vi "Autonomous Independent.vi"() -> ()   [LabVIEW 2015]
doc: "This VI is called when autonomous begins, and will automatically be terminated when autonomous ends. You can carry out timed or sensor driven robot movement independently without needing to return to the caller."
uses:
  <vilib>/Rock Robotics/WPI/CAN/TalonSRX/WPI_CANTalonSRX_BrakeOverride.ctl
  <vilib>/Rock Robotics/WPI/Utilities/WPI_GetSetVariantRefNum.vi
  <vilib>/Rock Robotics/Network Tables/NT Read String.vi
  <vilib>/Rock Robotics/Network Tables/NT Write Numeric Array.vi
  <vilib>/Rock Robotics/Network Tables/NT Write Number.vi
  <vilib>/addons/control/pid/pid.llb/PID (DBL).vi
  Robot Global Data.vi
  <vilib>/Rock Robotics/Network Tables/NT Read Number.vi
  <vilib>/addons/control/pid/NI_PID_pid.lvlib
  navX Library v2/navX Library v2.lvlib
panel:
  out "Shooter Output":dbl(graph)
  in  "Shoot Gains":T1={"proportional gain (Kc)"=1.0, "integral time (Ti, min)"=0.01, "derivative time (Td, min)"=0.0} {"derivative time (Td, min)" format="%.3f"; "integral time (Ti, min)" format="%.3f"; "proportional gain (Kc)" format="%.3f"}
  out "RPM":dbl(graph)
  in  "RPM 2":dbl
  in  "RPM":dbl
  in  "Aiming Gains":T1={"proportional gain (Kc)"=1.0, "integral time (Ti, min)"=0.01, "derivative time (Td, min)"=0.0} {"derivative time (Td, min)" format="%.3f"; "integral time (Ti, min)" format="%.3f"; "proportional gain (Kc)" format="%.3f"}
  out "Yaw":dbl(graph)
  in  "Target Angle":dbl=30.0
  out "E1 Rate":dbl
  out "E2 Rate":dbl
  out "Yaw Display":dbl
  in  "Single Turn Gains":T1={"proportional gain (Kc)"=0.12, "integral time (Ti, min)"=0.0, "derivative time (Td, min)"=0.0} {"derivative time (Td, min)" format="%.3f"; "integral time (Ti, min)" format="%.3f"; "proportional gain (Kc)" format="%.3f"}
  in  "Yaw":T1={"proportional gain (Kc)"=0.2, "integral time (Ti, min)"=0.0, "derivative time (Td, min)"=0.0} {"derivative time (Td, min)" format="%.3f"; "integral time (Ti, min)" format="%.3f"; "proportional gain (Kc)" format="%.3f"}
  out "Right Motor Speed":dbl(graph)
  out "Left Motor Speed":dbl(graph)
  out "Right Motor":dbl(graph)
  out "Left Motor":dbl(graph)
  in  "Distance":dbl=120.0
  in  "Speed Gains":T1={"proportional gain (Kc)"=0.65, "integral time (Ti, min)"=0.001, "derivative time (Td, min)"=0.001} {"derivative time (Td, min)" format="%.3f"; "integral time (Ti, min)" format="%.3f"; "proportional gain (Kc)" format="%.3f"}
  out "E2 Dist":dbl
  out "E1 Dist":dbl
  # "Be sure to right-click and choose Data Operations>>Make Current Value default if you want to save the array values with the VI"
  # "Encoder Distance Traveled"
  # "Speed we are assigning the motors and Encoder Rate"
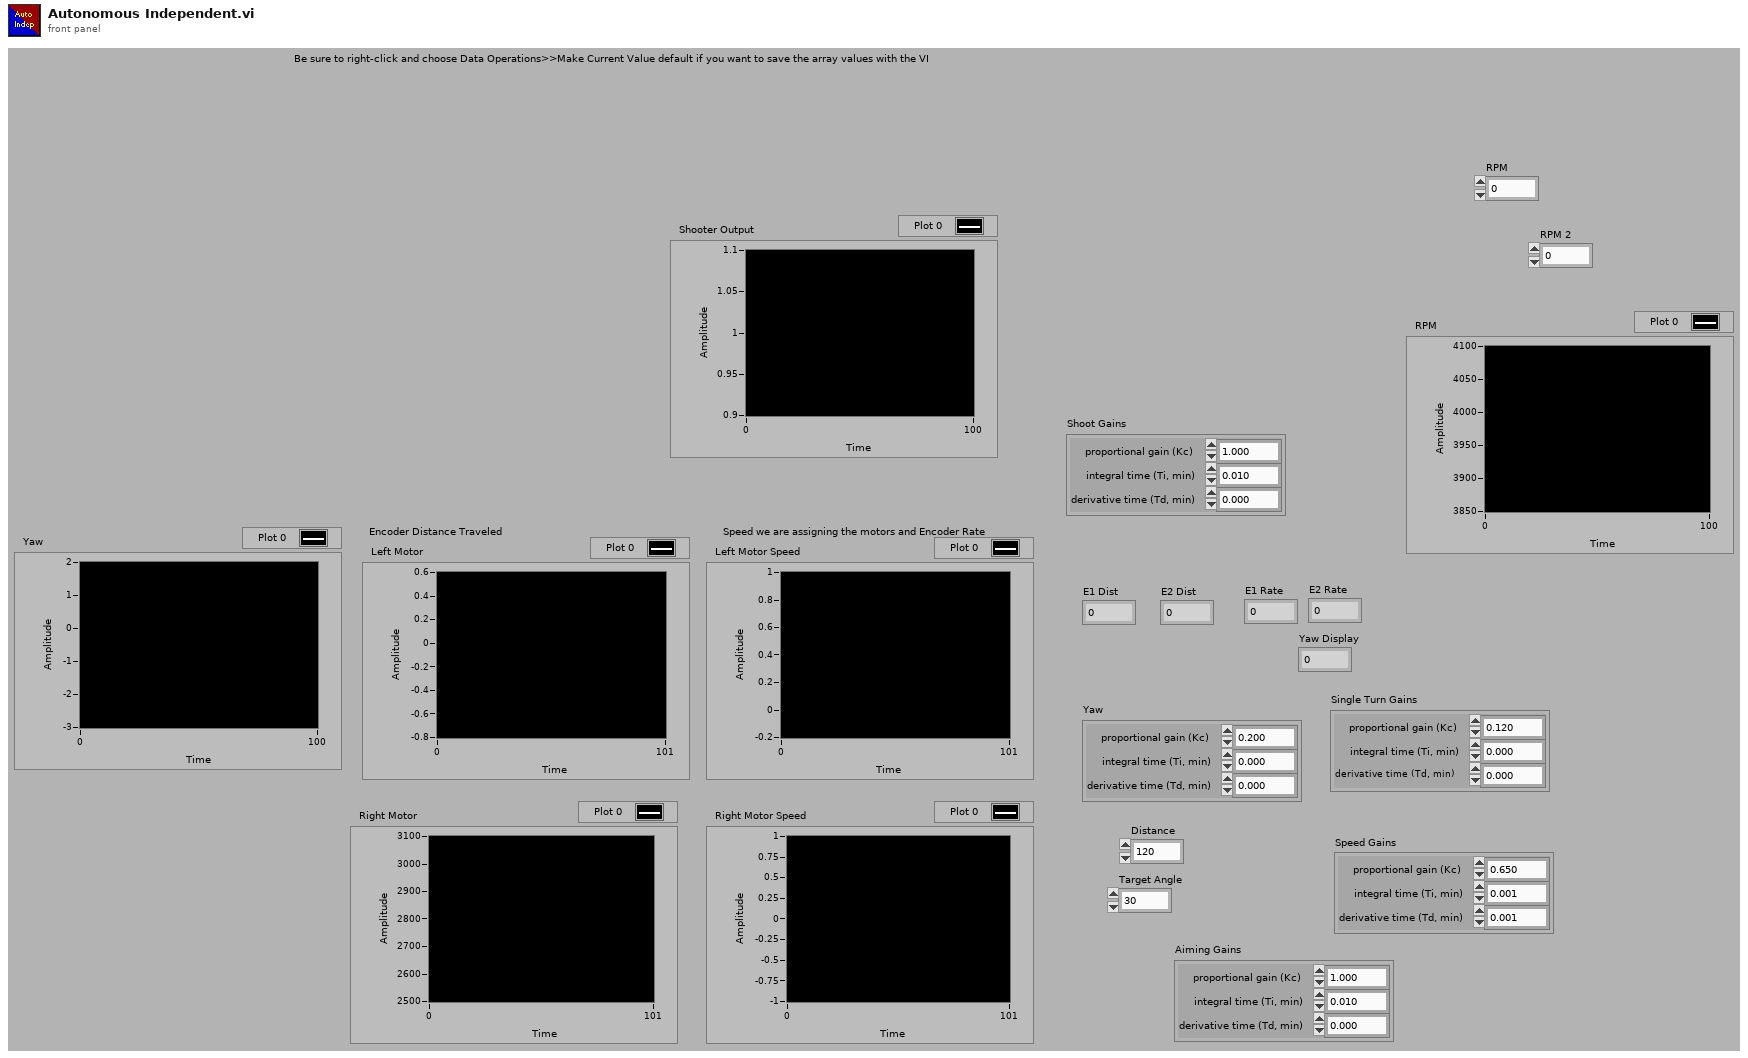
[diagram p1: front panel]
types:
  T1 = cluster{"proportional gain (Kc)":dbl, "integral time (Ti, min)":dbl, "derivative time (Td, min)":dbl}
  T2 = typedef "WPI_JoystickDevRef.ctl" = cluster{"Device":T3}
  T3 = typedef "WPI_JoystickDeviceEnum.ctl" = enum16{"USB 0", "USB 1", "USB 2", "USB 3", "USB 4", "USB 5"}
  T4 = typedef "WPI_CANTalonSRX_BrakeOverride.ctl" = enum8{"No Override", "Override to Coast", "Override to Brake"}
  T5 = typedef "navX Library v2.lvlib/Z900_navX_DeviceTypeDef.ctl" = cluster{"Interface":cluster{"Protocol":T6, "Update Rate (4Hz-60Hz)":u8, "navX Open TypeDef":variant}, "Notify Packet":refnum<notifier>, "Loop VI Refnum":refnum<vi>, "Ready to Close Occurrence Refnum":refnum<k4>}
  T6 = typedef "navX Library v2.lvlib/Z900_navX_ProtocolTypeDef.ctl" = enum16{"SERIAL", "I2C", "SPI"}
  T7 = typedef "WPI_EncoderDevRef.ctl" = cluster{"DevStatus":errorcluster, "EncoderIndex":T8, "CounterIndex":T9, "DistancePerCount":dbl, "Decoding Type":T10}
  T8 = typedef "FPGA_EncoderIdx.ctl" = enum8{"Enc 0", "Enc 1", "Enc 2", "Enc 3", "Enc 4", "Enc 5", "Enc 6", "Enc 7", "Invalid"}
  T9 = typedef "FPGA_CounterCtrSystemIndex.ctl" = enum8{"Ctr 0", "Ctr 1", "Ctr 2", "Ctr 3", "Ctr 4", "Ctr 5", "Ctr 6", "Ctr 7", "Invalid"}
  T10 = typedef "WPI_EncoderType.ctl" = enum16{"1x", "2x", "4x"}
  T11 = cluster{"Yaw":dbl, "Roll":dbl, "Pitch":dbl, "Heading":dbl, "Fused Heading":dbl}
  T12 = typedef "WPI_RobotDriveDevRef.ctl" = cluster{"DevStatus":errorcluster, "Motors[]":T13[], "Square Inputs":bool, "Max Output":dbl}
  T13 = typedef "WPI_MotorControlDeviceRef.ctl" = cluster{"DeviceStatus":errorcluster, "Type":T14, "PWM":cluster{"PWM Channel":T15, "DeadBand":T16}, "CAN":cluster{"Device Number":u8, "Control Mode":T17, "Semaphore":T18, "Max Vout":dbl, "TalonSRX Control Mode":T19}, "Invert":bool}
  T14 = typedef "WPI_MotorControlType.ctl" = enum16{"PWM", "CAN", "CANTalonSRX"}
  T15 = typedef "FPGA_DIOPWMChannel.ctl" = enum8{"PWM 0", "PWM 1", "PWM 2", "PWM 3", "PWM 4", "PWM 5", "PWM 6", "PWM 7", "PWM 8", "PWM 9", "PWM MXP 0", "PWM MXP 1", "PWM MXP 2", "PWM MXP 3", "PWM MXP 4", "PWM MXP 5", "PWM MXP 6", "PWM MXP 7", "PWM MXP 8", "PWM MXP 9", "Invalid"}
  T16 = typedef "WPI_PWMDeadband.ctl" = cluster{"Name":string, "maxPositivePwm":i32, "minPositivePwm":i32, "centerPwm":i32, "maxNegativePwm":i32, "minNegativePwm":i32, "angularRange":u16}
  T17 = typedef "WPI_CANJaguar_ControlMode.ctl" = enum8{"Percent VBus", "Current", "Speed", "Position", "Voltage"}
  T18 = typedef "Semaphore RefNum" = refnum<k1>
  T19 = typedef "WPI_CANTalonSRX_APIControlMode.ctl" = enum8{"Percent VBus", "Speed", "Position", "Slave", "Unchanged / Invalid", "Voltage Compensation", "Current", "Motion Profile"}
  T20 = typedef "WPI_CANTalonSRX_GlobalStatus.ctl" = cluster{"Applied Throttle":dbl, "Module Enabled":bool, "CAN Error":errorcluster, "Closed Loop Error":dbl, "Forward Limit Switch Closed":bool, "Reverse Limit Switch Closed":bool, "Sensor Position":dbl, "Sensor Velocity":dbl, "Current":dbl, "Sticky Fault - Over Temp":bool, "Sticky Fault - Under Voltage":bool, "Sticky Fault - Forward Limit":bool, "Sticky Fault - Reverse Limit":bool, "Sticky Fault - Forward Soft Limit":bool, "Sticky Fault - Reverse Soft Limit":bool, "Brake is Enabled":bool, "Encoder Position":dbl, "Encoder Velocity":dbl, "Encoder Index Count":dbl, "Encoder A Pin State":bool, "Encoder B Pin State":bool, "Encoder Index Pin State":bool, "Analog In":dbl, "Analog In Velocity":dbl, "Temperature (C)":dbl, "Battery Voltage":dbl, "Control 5 Is Supported":bool, "Current Profile Slot Select":dbl, "Pos Div 8":bool, "Vel Div 4":bool, "Pulse Width Position":i32, "Pulse Width Velocity":i32, "Pulse Width Rise To Rise (us)":i32, "Pulse Width Rise To Fall (us)":i32, "Mot Prof Active Is Under Run":bool, "Mot Prof Active Has Under Run":bool, "Mot Prof Active Is Last":bool, "Mot Prof Active Velocity Only":bool, "Mot Prof Active Is Valid":bool, "Mot Prof Buffer Is Full":bool, "Mot Prof Active Profile Slot Select":i32, "Mot Prof NextID":i32, "Mot Prof Count":i32, "Mot Prof Active Velocity":dbl, "Mot Prof Active Position":dbl, "Mot Prof Output Enable":i32}
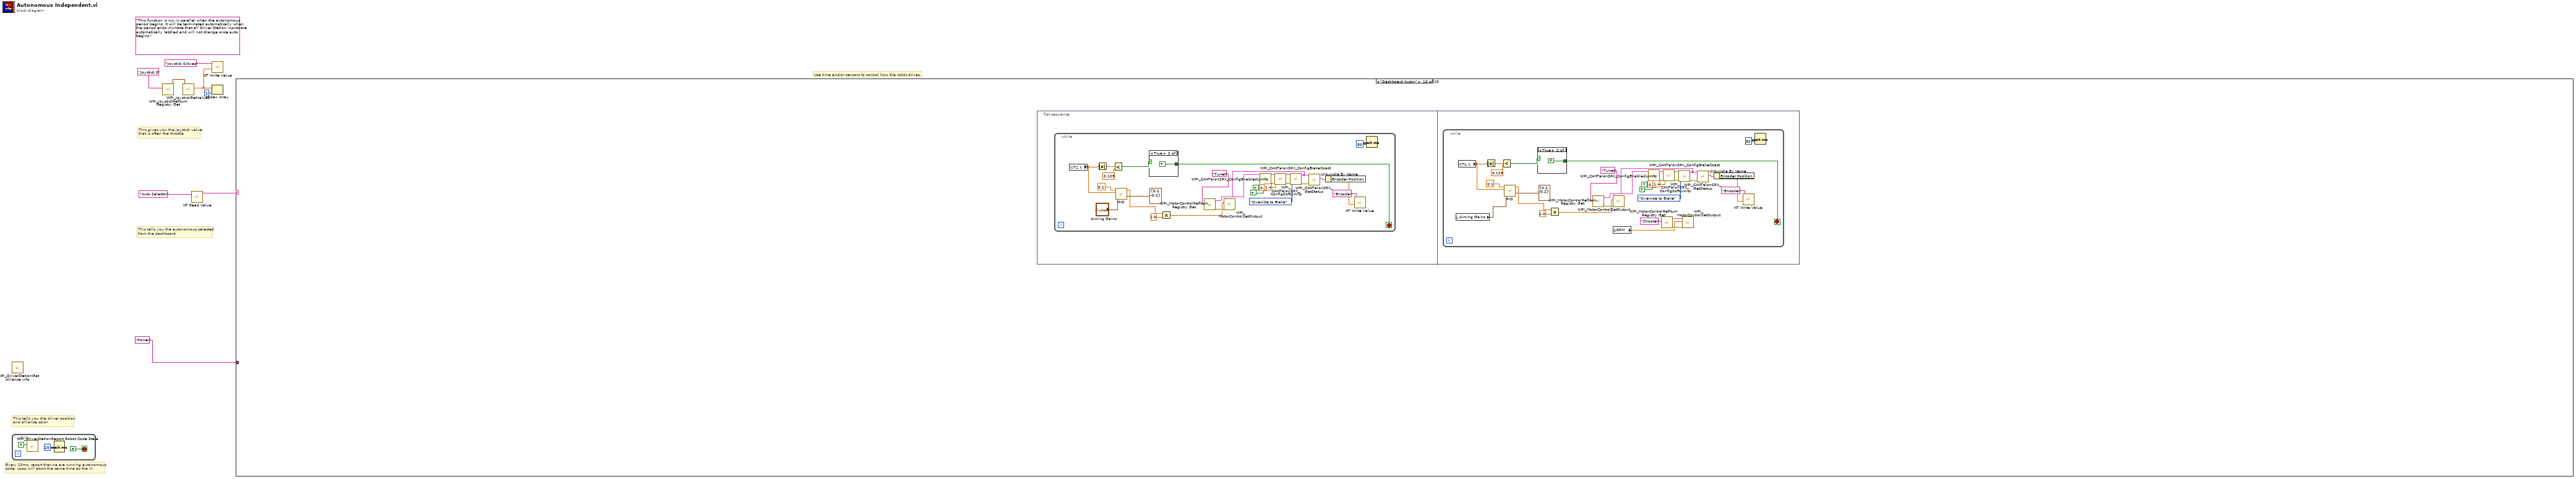
[diagram p0: block diagram]
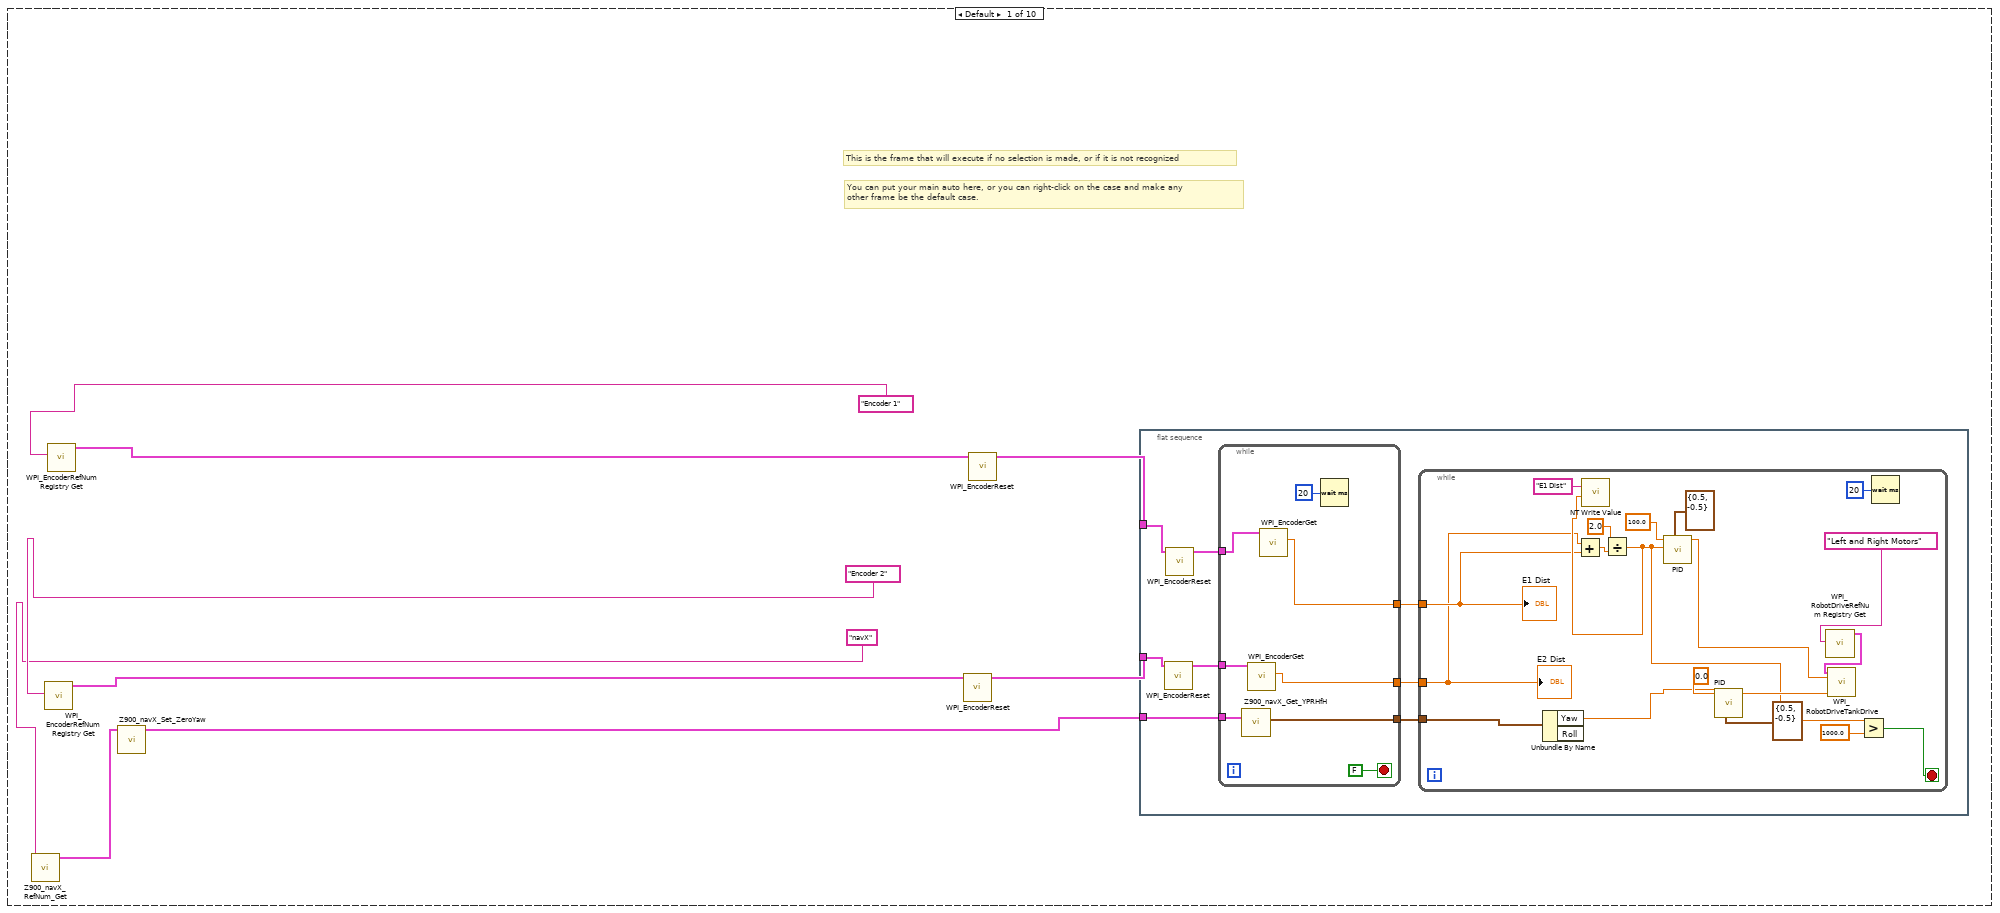
[diagram p2: hidden frame]
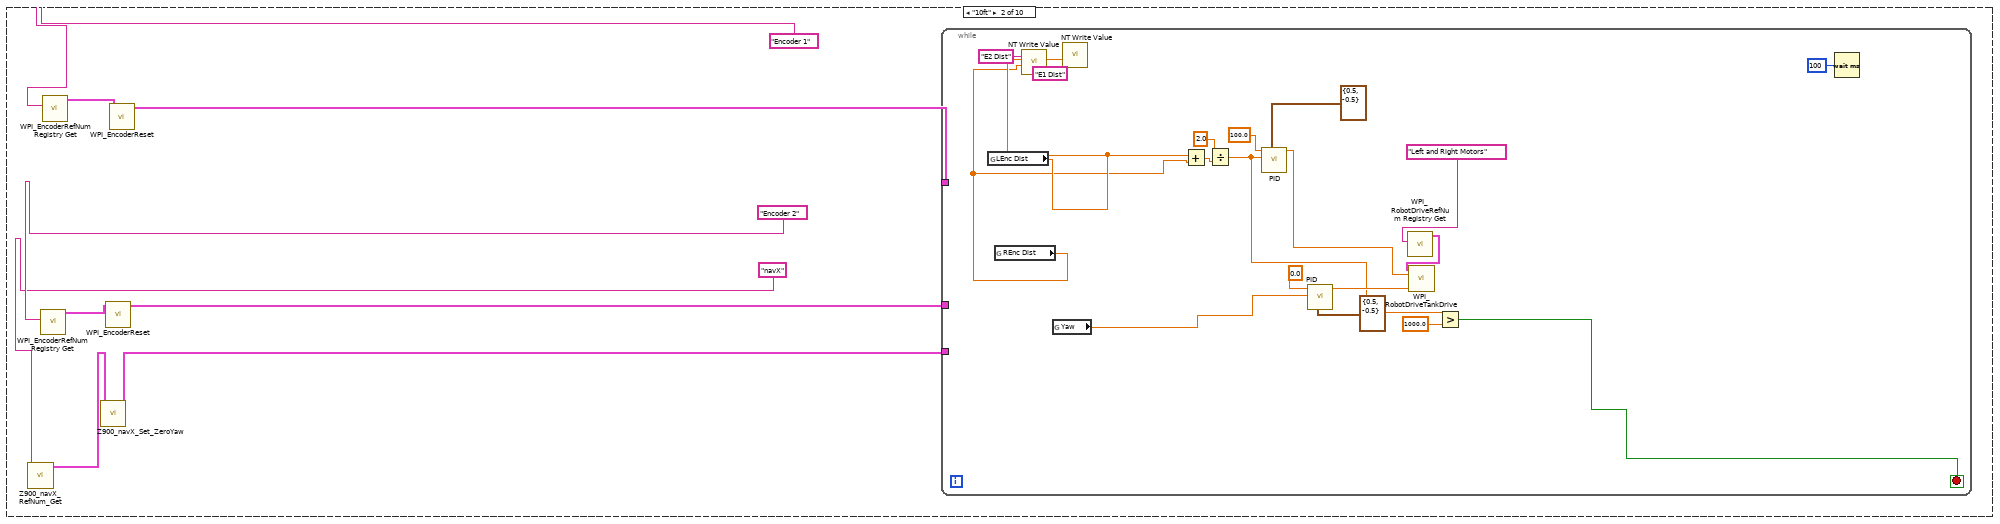
[diagram p3: hidden frame]
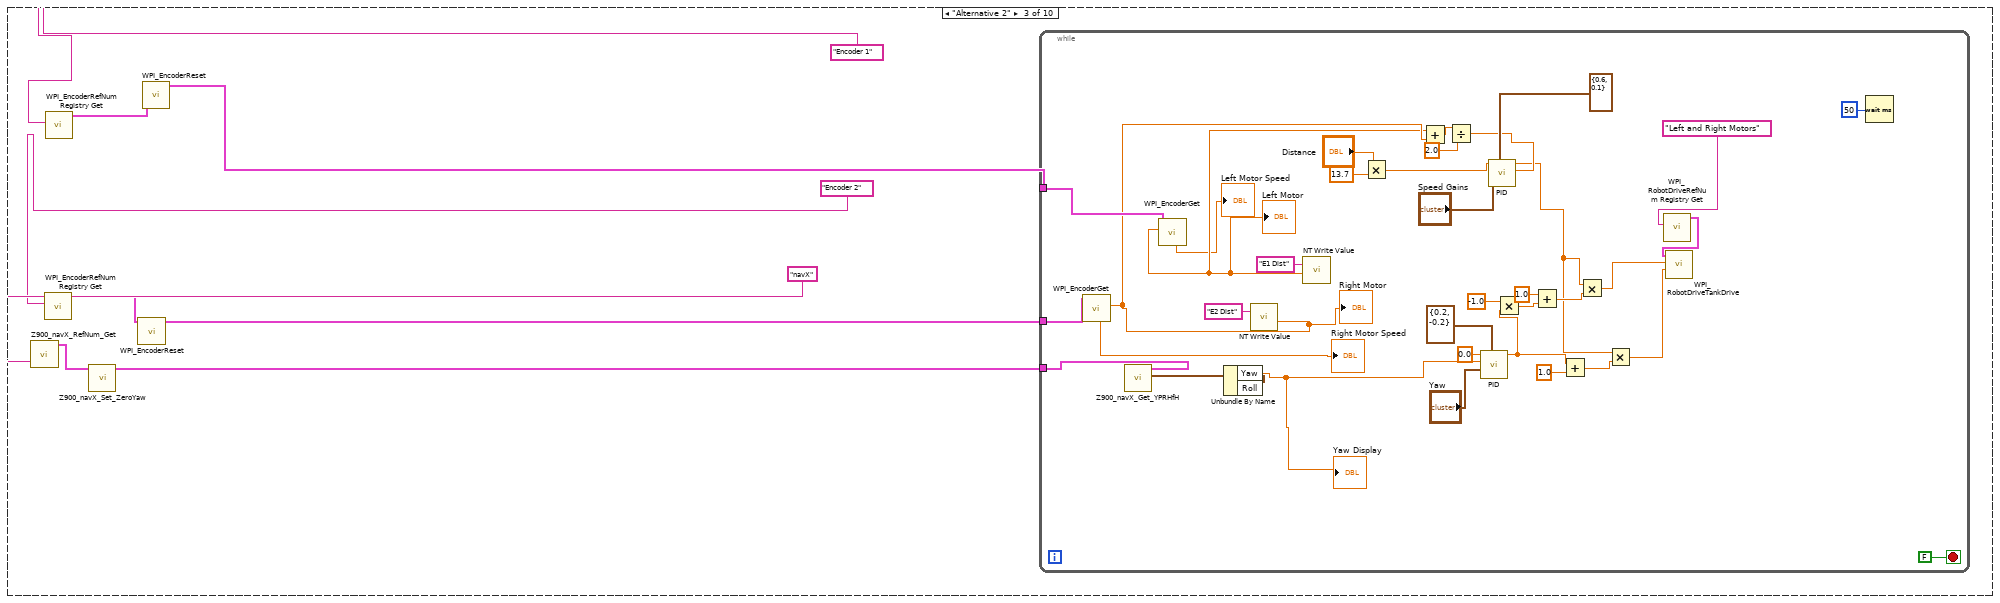
[diagram p4: hidden frame]
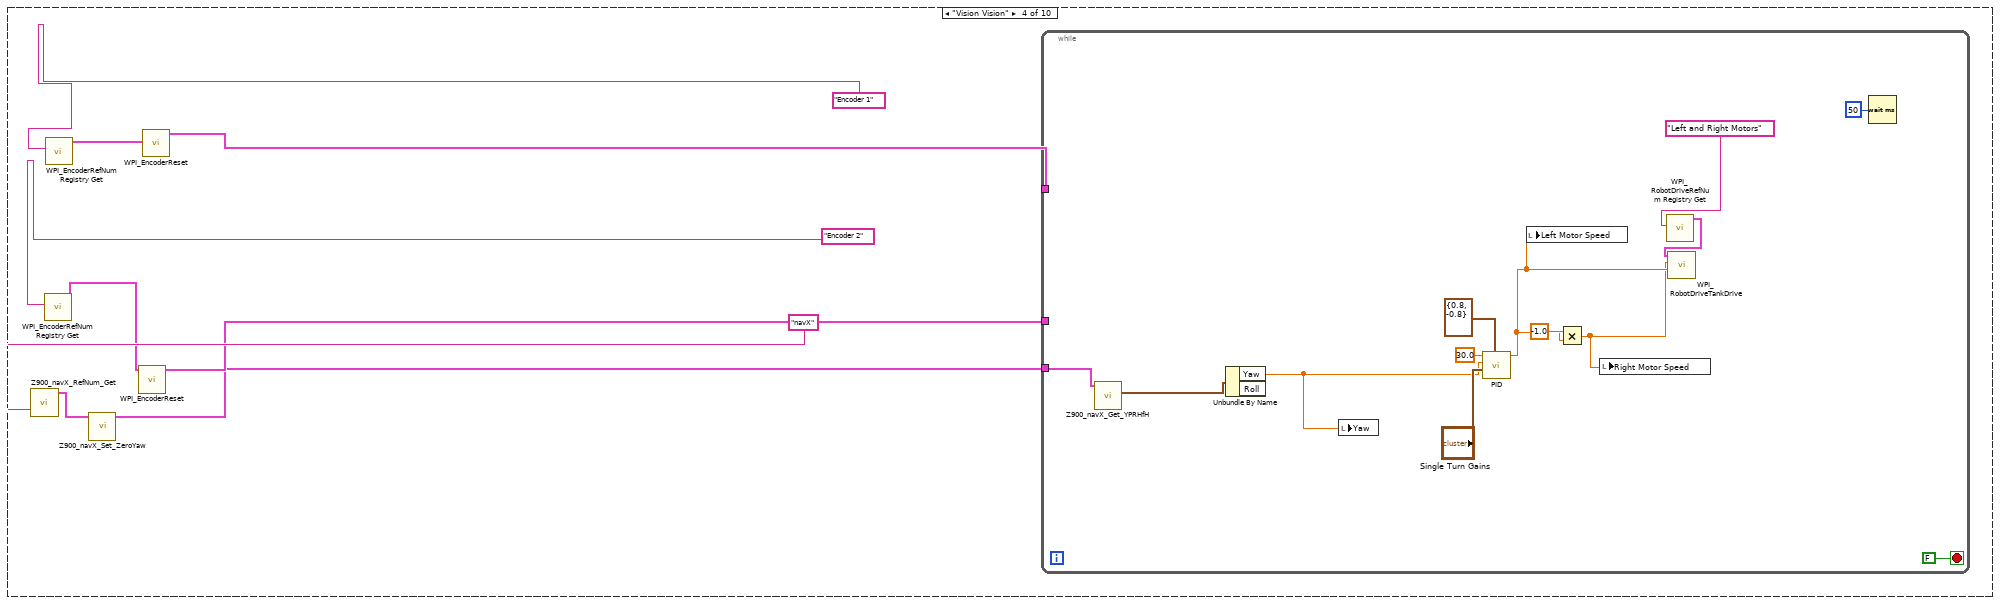
[diagram p5: hidden frame]
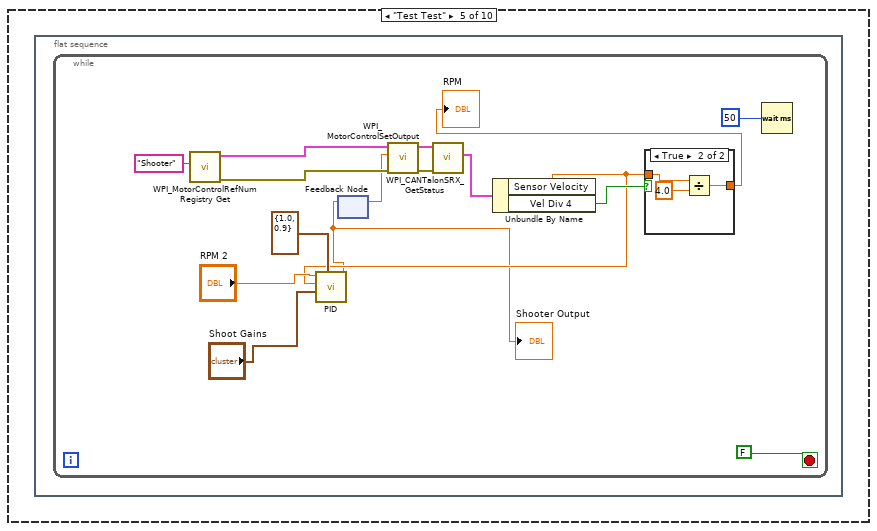
[diagram p6: hidden frame]
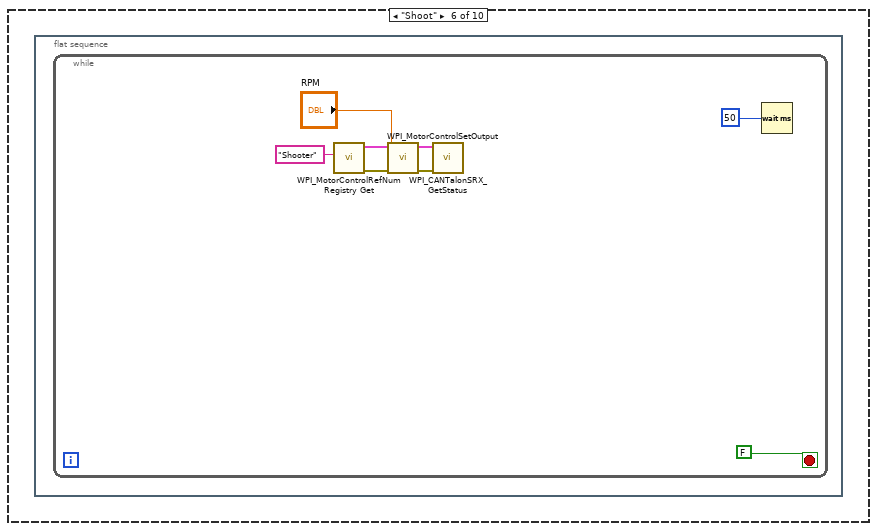
[diagram p8: hidden frame]
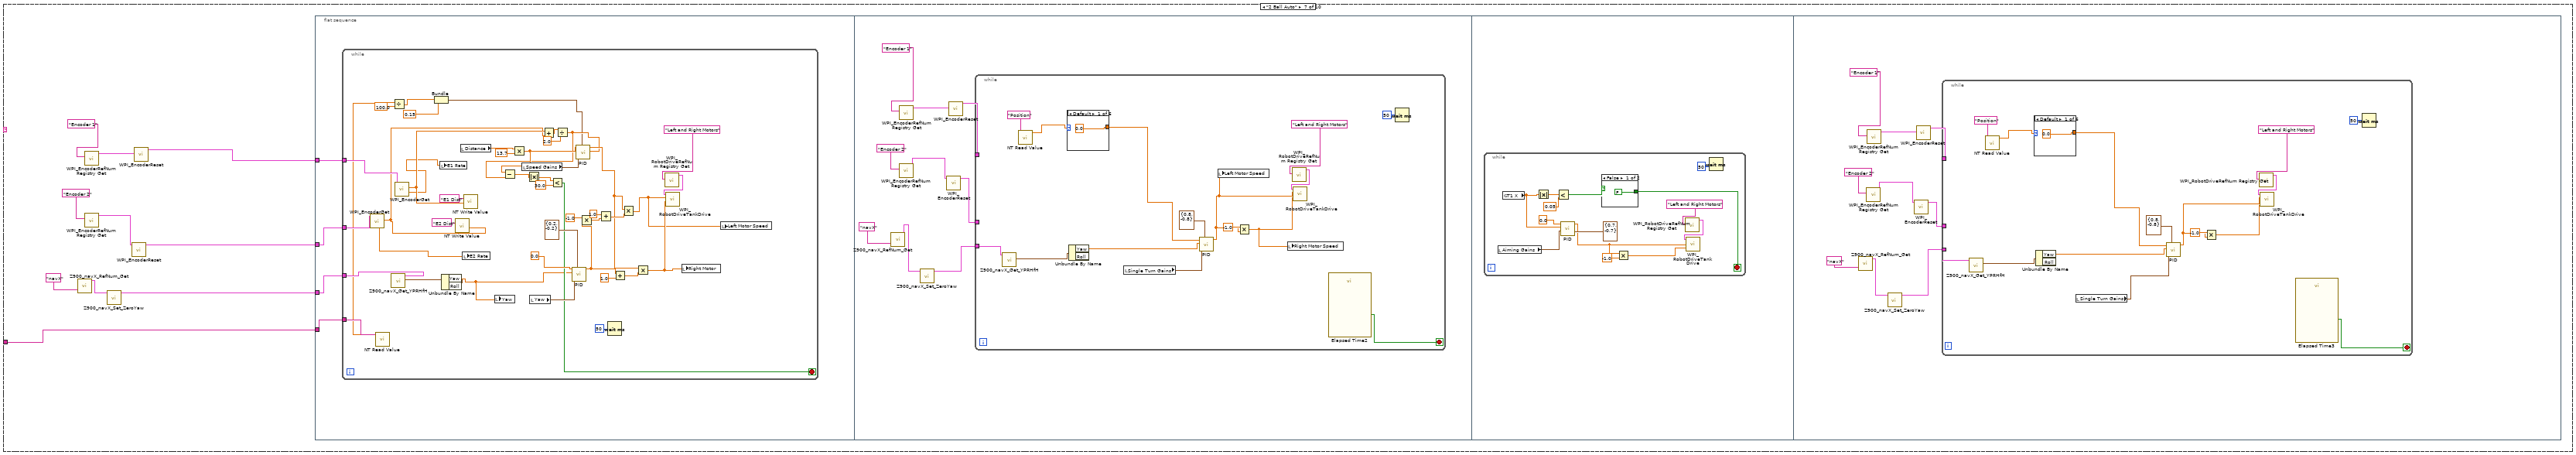
[diagram p9: hidden frame]
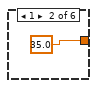
[diagram p10: hidden frame]
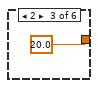
[diagram p11: hidden frame]
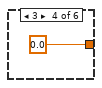
[diagram p12: hidden frame]
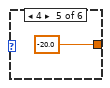
[diagram p13: hidden frame]
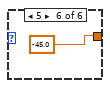
[diagram p14: hidden frame]
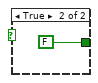
[diagram p15: hidden frame]
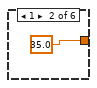
[diagram p16: hidden frame]
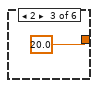
[diagram p17: hidden frame]
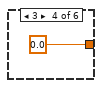
[diagram p18: hidden frame]
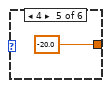
[diagram p19: hidden frame]
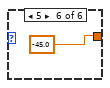
[diagram p20: hidden frame]
diagram:
  (unwired) "This function is run in parallel when the autonomous period begins. It will be terminated automatically when the period ends.\n\nNote that all Driver Station inputs are automatically latched and will not change once auto begins."
  # "This tells you the autonomous selected\nfrom the dashboard"
  # "Every 20ms, report that we are running autonomous\ncode. Loop will abort the same time as the VI."
  # "This gives you the joystick value\nthat is often the throttle"
  # "Use time and/or sensors to control how the robot drives."
  # "This tells you the driver position\nand alliance color"
  n1 = while {
    stop <- FALSE stop-if-true
    n2 = call <vilib>:"WPI_DriverStationReport Robot Code State.vi"("Autonomous"=TRUE) -> ()  [unwired: 10 in, 1 out]
    n3 = Wait (ms)(milliseconds to wait=u32 20) -> ()  [unwired: 1 out]
  }
  n4 = call <vilib>:"WPI_DriverStationGet Alliance Info.vi"() -> ()  [unwired: 12 out]
  n5 = call <vilib>:"WPI_JoystickRefNum Registry Get.vi"("refnum name"="Joystick 0") -> ("JoystickDevRef"=w7:T2)  [unwired: 1 in, 9 out]
  n6 = call <vilib>:"WPI_JoystickGetValues.vi"("JoystickDevRef"=w7) -> ("Axes"=w3:dbl[])  [unwired: 6 in, 4 out]
  n7 = call-poly <vilib>:"NT Read Value.vi"("Name"="Auto Selector") -> ("String"=w4:string)  [unwired: 9 in, 1 out]
  n8 = call-poly <vilib>:"NT Write Value.vi"("Numeric Array"=w3, "Name"="Joystick 0/Axes") -> ()  [unwired: 9 in, 1 out]
  n9 = Index Array(array=w3, index=2) -> ()  [unwired: 1 out]
  n10 = case shown="\"Dashboard Auton\"" w4 {
    tunnel: "Power" ("Name") -> [_ _ _ _ _ _ w179 _ w365 _]
    frame Default {
      # "You can put your main auto here, or you can right-click on the case and make any\nother frame be the default case."
      # "This is the frame that will execute if no selection is made, or if it is not recognized"
      n11 = call "Z900_navX_RefNum_Get.vi"("refnum name"="navX") -> ("navX Device"=w14:T5)  [unwired: 9 in, 1 out]
      n12 = call <vilib>:"WPI_EncoderRefNum Registry Get.vi"("refnum name"="Encoder 2") -> ("EncoderDevRef"=w16:T7)  [unwired: 9 in, 1 out]
      n13 = call <vilib>:"WPI_EncoderRefNum Registry Get.vi"("refnum name"="Encoder 1") -> ("EncoderDevRef"=w18:T7)  [unwired: 9 in, 1 out]
      n14 = call "Z900_navX_Set_ZeroYaw.vi"("navX Device"=w14) -> ("navX Device"=w13:T5)  [unwired: 9 in, 1 out]
      n15 = call <vilib>:"WPI_EncoderReset.vi"("EncoderDevRef"=w16) -> ("EncoderDevRef"=w15:T7)  [unwired: 9 in, 1 out]
      n16 = call <vilib>:"WPI_EncoderReset.vi"("EncoderDevRef"=w18) -> ("EncoderDevRef"=w17:T7)  [unwired: 9 in, 1 out]
      n17 = flat-sequence {
        tunnel: w17 -> [w28]
        tunnel: w15 -> [w27]
        tunnel: w13 -> [w26]
        frame #0 {
          n18 = call <vilib>:"WPI_EncoderReset.vi"("EncoderDevRef"=w27) -> ("EncoderDevRef"=w25:T7)  [unwired: 9 in, 1 out]
          n19 = call <vilib>:"WPI_EncoderReset.vi"("EncoderDevRef"=w28) -> ("EncoderDevRef"=w24:T7)  [unwired: 9 in, 1 out]
          n20 = while {
            tunnel: w26 -> [w33]
            tunnel: w25 -> [w34]
            tunnel: w24 -> [w35]
            tunnel: [w32] -> w23
            tunnel: [w31] -> w22
            tunnel: [w30] -> w21
            stop <- FALSE stop-if-true
            n21 = call "Z900_navX_Get_YPRHfH.vi"("navX Device"=w33) -> ("YRPHfH"=w32:T11)  [unwired: 7 in, 3 out]
            n22 = call <vilib>:"WPI_EncoderGet.vi"("EncoderDevRef"=w34) -> ("Distance"=w31:dbl)  [unwired: 5 in, 5 out]
            n23 = call <vilib>:"WPI_EncoderGet.vi"("EncoderDevRef"=w35) -> ("Distance"=w30:dbl)  [unwired: 5 in, 5 out]
            n24 = Wait (ms)(milliseconds to wait=u32 20) -> ()  [unwired: 1 out]
          }
          n25 = while {
            tunnel: w23 -> [w40]
            tunnel: w22 -> [w38]
            tunnel: w21 -> [w39]
            stop <- w44 stop-if-true
            n26 = Unbundle By Name(w40) -> ("Yaw"=w41:dbl)  [unwired: 1 out]
            n27 = Add(x=w38, y=w39) -> (x+y=w55:dbl)
            n28 = Divide(x=2.0, y=w55) -> (x/y=w43:dbl)
            n29 = call-poly <vilib>:"NT Write Value.vi"("Numeric"=w43, "Name"="E1 Dist") -> ()  [unwired: 9 in, 1 out]
            n30 = call-poly <vilib>:"PID.vi"("output range"=cluster{"output high":dbl, "output low":dbl} {"output high"=0.5, "output low"=-0.5}, "process variable"=w43, "setpoint"=100.0) -> ("output"=w48:dbl)  [unwired: 7 in, 1 out]
            n31 = call-poly <vilib>:"PID.vi"("output range"=cluster{"output high":dbl, "output low":dbl} {"output high"=0.5, "output low"=-0.5}, "process variable"=w41, "setpoint"=0.0) -> ("output"=w47:dbl)  [unwired: 7 in, 1 out]
            n32 = call <vilib>:"WPI_RobotDriveRefNum Registry Get.vi"("refnum name"="Left and Right Motors") -> ("RobotDriveDevRef"=w50:T12)  [unwired: 9 in, 1 out]
            n33 = call <vilib>:"WPI_RobotDriveTankDrive.vi"("Right axis value"=w47, "Left axis value"=w48, "RobotDriveDevRef"=w50) -> ()  [unwired: 6 in, 3 out]
            n34 = Greater?(x=w43, y=1000.0) -> (0:w44:bool)
            n35 = Wait (ms)(milliseconds to wait=u32 20) -> ()  [unwired: 1 out]
            "E2 Dist" <- w38
            "E1 Dist" <- w39
          }
        }
      }
    }
    frame "10ft" {
      n36 = call "Z900_navX_RefNum_Get.vi"("refnum name"="navX") -> ("navX Device"=w58:T5)  [unwired: 9 in, 1 out]
      n37 = call <vilib>:"WPI_EncoderRefNum Registry Get.vi"("refnum name"="Encoder 2") -> ("EncoderDevRef"=w60:T7)  [unwired: 9 in, 1 out]
      n38 = call <vilib>:"WPI_EncoderRefNum Registry Get.vi"("refnum name"="Encoder 1") -> ("EncoderDevRef"=w62:T7)  [unwired: 9 in, 1 out]
      n39 = call "Z900_navX_Set_ZeroYaw.vi"("navX Device"=w58) -> ("navX Device"=w57:T5)  [unwired: 9 in, 1 out]
      n40 = call <vilib>:"WPI_EncoderReset.vi"("EncoderDevRef"=w60) -> ("EncoderDevRef"=w59:T7)  [unwired: 9 in, 1 out]
      n41 = call <vilib>:"WPI_EncoderReset.vi"("EncoderDevRef"=w62) -> ("EncoderDevRef"=w61:T7)  [unwired: 9 in, 1 out]
      n42 = while {
        tunnel: w61 -> [_]
        tunnel: w59 -> [_]
        tunnel: w57 -> [_]
        stop <- w65 stop-if-true
        n43 = global read "Robot Global Data.vi" "LEnc Dist"() -> (w68:dbl)
        n44 = global read "Robot Global Data.vi" "REnc Dist"() -> (w67:dbl)
        n45 = call-poly <vilib>:"NT Write Value.vi"("Numeric"=w67, "Name"="E2 Dist") -> ()  [unwired: 9 in, 1 out]
        n46 = global read "Robot Global Data.vi" "Yaw"() -> (w66:dbl)
        n47 = call-poly <vilib>:"NT Write Value.vi"("Numeric"=w68, "Name"="E1 Dist") -> ()  [unwired: 9 in, 1 out]
        n48 = Add(x=w68, y=w67) -> (x+y=w82:dbl)
        n49 = Divide(x=2.0, y=w82) -> (x/y=w72:dbl)
        n50 = call-poly <vilib>:"PID.vi"("output range"=cluster{"output high":dbl, "output low":dbl} {"output high"=0.5, "output low"=-0.5}, "process variable"=w72, "setpoint"=100.0) -> ("output"=w76:dbl)  [unwired: 7 in, 1 out]
        n51 = call-poly <vilib>:"PID.vi"("output range"=cluster{"output high":dbl, "output low":dbl} {"output high"=0.5, "output low"=-0.5}, "process variable"=w66, "setpoint"=0.0) -> ("output"=w75:dbl)  [unwired: 7 in, 1 out]
        n52 = call <vilib>:"WPI_RobotDriveRefNum Registry Get.vi"("refnum name"="Left and Right Motors") -> ("RobotDriveDevRef"=w78:T12)  [unwired: 9 in, 1 out]
        n53 = call <vilib>:"WPI_RobotDriveTankDrive.vi"("Right axis value"=w75, "Left axis value"=w76, "RobotDriveDevRef"=w78) -> ()  [unwired: 6 in, 3 out]
        n54 = Greater?(x=w72, y=1000.0) -> (0:w65:bool)
        n55 = Wait (ms)(milliseconds to wait=u32 100) -> ()  [unwired: 1 out]
      }
    }
    frame "Alternative 2" {
      n56 = call "Z900_navX_RefNum_Get.vi"("refnum name"="navX") -> ("navX Device"=w85:T5)  [unwired: 9 in, 1 out]
      n57 = call <vilib>:"WPI_EncoderRefNum Registry Get.vi"("refnum name"="Encoder 2") -> ("EncoderDevRef"=w87:T7)  [unwired: 9 in, 1 out]
      n58 = call <vilib>:"WPI_EncoderRefNum Registry Get.vi"("refnum name"="Encoder 1") -> ("EncoderDevRef"=w89:T7)  [unwired: 9 in, 1 out]
      n59 = call "Z900_navX_Set_ZeroYaw.vi"("navX Device"=w85) -> ("navX Device"=w84:T5)  [unwired: 9 in, 1 out]
      n60 = call <vilib>:"WPI_EncoderReset.vi"("EncoderDevRef"=w87) -> ("EncoderDevRef"=w86:T7)  [unwired: 9 in, 1 out]
      n61 = call <vilib>:"WPI_EncoderReset.vi"("EncoderDevRef"=w89) -> ("EncoderDevRef"=w88:T7)  [unwired: 9 in, 1 out]
      n62 = while {
        tunnel: w88 -> [w121]
        tunnel: w86 -> [w120]
        tunnel: w84 -> [w119]
        stop <- FALSE stop-if-true
        n63 = call <vilib>:"WPI_EncoderGet.vi"("EncoderDevRef"=w120) -> ("Distance"=w110:dbl, "Rate"=→"Right Motor Speed":dbl)  [unwired: 5 in, 4 out]
        "Right Motor" <- w110
        n64 = call "Z900_navX_Get_YPRHfH.vi"("navX Device"=w119) -> ("YRPHfH"=w122:T11)  [unwired: 7 in, 3 out]
        n65 = call <vilib>:"WPI_EncoderGet.vi"("EncoderDevRef"=w121) -> ("Distance"=w109:dbl, "Rate"=→"Left Motor Speed":dbl)  [unwired: 5 in, 4 out]
        "Left Motor" <- w109
        n66 = Unbundle By Name(w122) -> ("Yaw"=w95:dbl)  [unwired: 1 out]
        "Yaw Display" <- w95
        n67 = call-poly <vilib>:"NT Write Value.vi"("Numeric"=w110, "Name"="E2 Dist") -> ()  [unwired: 9 in, 1 out]
        n68 = call-poly <vilib>:"NT Write Value.vi"("Numeric"=w109, "Name"="E1 Dist") -> ()  [unwired: 9 in, 1 out]
        n69 = Multiply(x="Distance", y=13.7) -> (x*y=w111:dbl)
        n70 = Add(x=w109, y=w110) -> (x+y=w116:dbl)
        n71 = Divide(x=w116, y=2.0) -> (x/y=w114:dbl)
        n72 = call-poly <vilib>:"PID.vi"("output range"=cluster{"output high":dbl, "output low":dbl} {"output high"=0.2, "output low"=-0.2}, "PID gains"="Yaw", "process variable"=w95, "setpoint"=0.0) -> ("output"=w99:dbl)  [unwired: 6 in, 1 out]
        n73 = call-poly <vilib>:"PID.vi"("output range"=cluster{"output high":dbl, "output low":dbl} {"output high"=0.6, "output low"=0.1}, "PID gains"="Speed Gains", "process variable"=w114, "setpoint"=w111) -> ("output"=w96:dbl)  [unwired: 6 in, 1 out]
        n74 = Multiply(x=-1.0, y=w99) -> (x*y=w100:dbl)
        n75 = Add(x=1.0, y=w100) -> (x+y=w101:dbl)
        n76 = Add(x=w99, y=1.0) -> (x+y=w102:dbl)
        n77 = Multiply(x=w96, y=w101) -> (x*y=w93:dbl)
        n78 = Multiply(x=w96, y=w102) -> (x*y=w94:dbl)
        n79 = call <vilib>:"WPI_RobotDriveRefNum Registry Get.vi"("refnum name"="Left and Right Motors") -> ("RobotDriveDevRef"=w124:T12)  [unwired: 9 in, 1 out]
        n80 = call <vilib>:"WPI_RobotDriveTankDrive.vi"("Right axis value"=w94, "Left axis value"=w93, "RobotDriveDevRef"=w124) -> ()  [unwired: 6 in, 3 out]
        n81 = Wait (ms)(milliseconds to wait=u32 50) -> ()  [unwired: 1 out]
      }
    }
    frame "Vision Vision" {
      n82 = call "Z900_navX_RefNum_Get.vi"("refnum name"="navX") -> ("navX Device"=w130:T5)  [unwired: 9 in, 1 out]
      n83 = call <vilib>:"WPI_EncoderRefNum Registry Get.vi"("refnum name"="Encoder 2") -> ("EncoderDevRef"=w132:T7)  [unwired: 9 in, 1 out]
      n84 = call <vilib>:"WPI_EncoderRefNum Registry Get.vi"("refnum name"="Encoder 1") -> ("EncoderDevRef"=w134:T7)  [unwired: 9 in, 1 out]
      n85 = call "Z900_navX_Set_ZeroYaw.vi"("navX Device"=w130) -> ("navX Device"=w129:T5)  [unwired: 9 in, 1 out]
      n86 = call <vilib>:"WPI_EncoderReset.vi"("EncoderDevRef"=w132) -> ("EncoderDevRef"=w131:T7)  [unwired: 9 in, 1 out]
      n87 = call <vilib>:"WPI_EncoderReset.vi"("EncoderDevRef"=w134) -> ("EncoderDevRef"=w133:T7)  [unwired: 9 in, 1 out]
      n88 = while {
        tunnel: w133 -> [_]
        tunnel: w131 -> [_]
        tunnel: w129 -> [w144]
        stop <- FALSE stop-if-true
        n89 = call "Z900_navX_Get_YPRHfH.vi"("navX Device"=w144) -> ("YRPHfH"=w143:T11)  [unwired: 7 in, 3 out]
        n90 = Unbundle By Name(w143) -> ("Yaw"=w138:dbl)  [unwired: 1 out]
        n91 = local write "Yaw"(w138) -> ()
        n92 = call-poly <vilib>:"PID.vi"("output range"=cluster{"output high":dbl, "output low":dbl} {"output high"=0.8, "output low"=-0.8}, "PID gains"="Single Turn Gains", "process variable"=w138, "setpoint"=30.0) -> ("output"=w140:dbl)  [unwired: 6 in, 1 out]
        n93 = local write "Left Motor Speed"(w140) -> ()
        n94 = Multiply(x=-1.0, y=w140) -> (x*y=w139:dbl)
        n95 = local write "Right Motor Speed"(w139) -> ()
        n96 = call <vilib>:"WPI_RobotDriveRefNum Registry Get.vi"("refnum name"="Left and Right Motors") -> ("RobotDriveDevRef"=w149:T12)  [unwired: 9 in, 1 out]
        n97 = call <vilib>:"WPI_RobotDriveTankDrive.vi"("Right axis value"=w140, "Left axis value"=w139, "RobotDriveDevRef"=w149) -> ()  [unwired: 6 in, 3 out]
        n98 = Wait (ms)(milliseconds to wait=u32 50) -> ()  [unwired: 1 out]
      }
    }
    frame "Test Test" {
      n99 = flat-sequence {
        frame #0 {
          n100 = while {
            stop <- FALSE stop-if-true
            n101 = call <vilib>:"WPI_MotorControlRefNum Registry Get.vi"("refnum name"="Shooter") -> ("error out"=w166:errorcluster, "MotorControlDevRef"=w165:T13)  [unwired: 9 in]
            n102 = feedback #1() -> (w152:dbl)  [unwired: 1 in]
            n103 = call <vilib>:"WPI_MotorControlSetOutput.vi"("error in (no error)"=w166, "Output"=w152, "MotorControlDevRef"=w165) -> ("error out"=w163:errorcluster, "MotorControlDevRef"=w162:T13)  [unwired: 6 in, 1 out]
            n104 = call <vilib>:"WPI_CANTalonSRX_GetStatus.vi"("error in (no error)"=w163, "CAN Talon SRX Ref"=w162) -> ("Talon SRX Status"=w159:T20)  [unwired: 7 in, 2 out]
            n105 = Unbundle By Name(w159) -> ("Sensor Velocity"=w154:dbl, "Vel Div 4"=w158:bool)
            n106 = call-poly <vilib>:"PID.vi"("output range"=cluster{"output high":dbl, "output low":dbl} {"output high"=1.0, "output low"=0.9}, "PID gains"="Shoot Gains", "process variable"=w154, "setpoint"="RPM 2") -> ("output"=w151:dbl)  [unwired: 6 in, 1 out]
            "Shooter Output" <- w151
            n107 = feedback-in #1(w151) -> ()
            n108 = case shown="True" w158 {
              tunnel: w154 -> [w167 w170]
              tunnel: [w167 w168] -> w157
              frame False {
              }
              frame True {
                n109 = Divide(x=w170, y=4.0) -> (x/y=w168:dbl)
              }
            }
            "RPM" <- w157
            n110 = Wait (ms)(milliseconds to wait=50) -> ()  [unwired: 1 out]
          }
        }
      }
    }
    frame "Shoot" {
      n111 = flat-sequence {
        frame #0 {
          n112 = while {
            stop <- FALSE stop-if-true
            n113 = call <vilib>:"WPI_MotorControlRefNum Registry Get.vi"("refnum name"="Shooter") -> ("error out"=w178:errorcluster, "MotorControlDevRef"=w177:T13)  [unwired: 9 in]
            n114 = call <vilib>:"WPI_MotorControlSetOutput.vi"("error in (no error)"=w178, "Output"="RPM", "MotorControlDevRef"=w177) -> ("error out"=w175:errorcluster, "MotorControlDevRef"=w174:T13)  [unwired: 6 in, 1 out]
            n115 = call <vilib>:"WPI_CANTalonSRX_GetStatus.vi"("error in (no error)"=w175, "CAN Talon SRX Ref"=w174) -> ()  [unwired: 7 in, 3 out]
            n116 = Wait (ms)(milliseconds to wait=50) -> ()  [unwired: 1 out]
          }
        }
      }
    }
    frame "2 Ball Auto" {
      n117 = call "Z900_navX_RefNum_Get.vi"("refnum name"="navX") -> ("navX Device"=w187:T5)  [unwired: 9 in, 1 out]
      n118 = call <vilib>:"WPI_EncoderRefNum Registry Get.vi"("refnum name"="Encoder 2") -> ("EncoderDevRef"=w185:T7)  [unwired: 9 in, 1 out]
      n119 = call <vilib>:"WPI_EncoderRefNum Registry Get.vi"("refnum name"="Encoder 1") -> ("EncoderDevRef"=w183:T7)  [unwired: 9 in, 1 out]
      n120 = call "Z900_navX_Set_ZeroYaw.vi"("navX Device"=w187) -> ("navX Device"=w188:T5)  [unwired: 9 in, 1 out]
      n121 = call <vilib>:"WPI_EncoderReset.vi"("EncoderDevRef"=w185) -> ("EncoderDevRef"=w186:T7)  [unwired: 9 in, 1 out]
      n122 = call <vilib>:"WPI_EncoderReset.vi"("EncoderDevRef"=w183) -> ("EncoderDevRef"=w184:T7)  [unwired: 9 in, 1 out]
      n123 = flat-sequence {
        tunnel: w188 -> [w192]
        tunnel: w186 -> [w191]
        tunnel: w184 -> [w190]
        tunnel: w179 -> [w189]
        frame #0 {
          n124 = while {
            tunnel: w190 -> [w230]
            tunnel: w191 -> [w229]
            tunnel: w192 -> [w228]
            tunnel: w189 -> [w202]
            stop <- w203 stop-if-true
            n125 = call <vilib>:"WPI_EncoderGet.vi"("EncoderDevRef"=w229) -> ("Distance"=w209:dbl, "Rate"=w194:dbl)  [unwired: 5 in, 4 out]
            n126 = call-poly <vilib>:"NT Read Value.vi"("Name"=w202) -> ("Numeric"=w201:dbl)  [unwired: 9 in, 1 out]
            n127 = call "Z900_navX_Get_YPRHfH.vi"("navX Device"=w228) -> ("YRPHfH"=w231:T11)  [unwired: 7 in, 3 out]
            n128 = Divide(x=w201, y=100.0) -> (x/y=w199:dbl)
            n129 = call <vilib>:"WPI_EncoderGet.vi"("EncoderDevRef"=w230) -> ("Distance"=w210:dbl, "Rate"=w193:dbl)  [unwired: 5 in, 4 out]
            n130 = Bundle(w199, "output low"=0.15) -> (w197:cluster{dbl, "output low":dbl})  [unwired: 1 in]
            n131 = local write "E1 Rate"(w193) -> ()
            n132 = Unbundle By Name(w231) -> ("Yaw"=w195:dbl)  [unwired: 1 out]
            n133 = call-poly <vilib>:"NT Write Value.vi"("Numeric"=w209, "Name"="E2 Dist") -> ()  [unwired: 9 in, 1 out]
            n134 = local read "Distance"() -> (w196:dbl)
            n135 = local write "E2 Rate"(w194) -> ()
            n136 = call-poly <vilib>:"NT Write Value.vi"("Numeric"=w210, "Name"="E1 Dist") -> ()  [unwired: 9 in, 1 out]
            n137 = local write "Yaw"(w195) -> ()
            n138 = Multiply(x=w196, y=13.7) -> (x*y=w208:dbl)
            n139 = local read "Speed Gains"() -> (w212:T1)
            n140 = local read "Yaw"() -> (w215:T1)
            n141 = Add(x=w210, y=w209) -> (x+y=w227:dbl)
            n142 = Divide(x=w227, y=2.0) -> (x/y=w207:dbl)
            n143 = Subtract(x=w208, y=w207) -> (x-y=w206:dbl)
            n144 = Absolute Value(x=w206) -> (abs(x)=w205:dbl)
            n145 = Less?(x=w205, y=30.0) -> (x < y?=w203:bool)
            n146 = call-poly <vilib>:"PID.vi"("output range"=cluster{"output high":dbl, "output low":dbl} {"output high"=0.2, "output low"=-0.2}, "PID gains"=w215, "process variable"=w195, "setpoint"=0.0) -> ("output"=w220:dbl)  [unwired: 6 in, 1 out]
            n147 = call-poly <vilib>:"PID.vi"("output range"=w197, "PID gains"=w212, "process variable"=w207, "setpoint"=w208) -> ("output"=w217:dbl)  [unwired: 6 in, 1 out]
            n148 = Multiply(x=-1.0, y=w220) -> (x*y=w221:dbl)
            n149 = Add(x=1.0, y=w221) -> (x+y=w222:dbl)
            n150 = Wait (ms)(milliseconds to wait=u32 50) -> ()  [unwired: 1 out]
            n151 = Add(x=w220, y=1.0) -> (x+y=w223:dbl)
            n152 = Multiply(x=w217, y=w222) -> (x*y=w213:dbl)
            n153 = Multiply(x=w217, y=w223) -> (x*y=w214:dbl)
            n154 = call <vilib>:"WPI_RobotDriveRefNum Registry Get.vi"("refnum name"="Left and Right Motors") -> ("RobotDriveDevRef"=w233:T12)  [unwired: 9 in, 1 out]
            n155 = call <vilib>:"WPI_RobotDriveTankDrive.vi"("Right axis value"=w214, "Left axis value"=w213, "RobotDriveDevRef"=w233) -> ()  [unwired: 6 in, 3 out]
            n156 = local write "Right Motor"(w214) -> ()
            n157 = local write "Left Motor Speed"(w213) -> ()
          }
        }
        frame #1 {
          n158 = call "Z900_navX_RefNum_Get.vi"("refnum name"="navX") -> ("navX Device"=w238:T5)  [unwired: 9 in, 1 out]
          n159 = call <vilib>:"WPI_EncoderRefNum Registry Get.vi"("refnum name"="Encoder 2") -> ("EncoderDevRef"=w240:T7)  [unwired: 9 in, 1 out]
          n160 = call <vilib>:"WPI_EncoderRefNum Registry Get.vi"("refnum name"="Encoder 1") -> ("EncoderDevRef"=w242:T7)  [unwired: 9 in, 1 out]
          n161 = call "Z900_navX_Set_ZeroYaw.vi"("navX Device"=w238) -> ("navX Device"=w237:T5)  [unwired: 9 in, 1 out]
          n162 = call <vilib>:"WPI_EncoderReset.vi"("EncoderDevRef"=w240) -> ("EncoderDevRef"=w239:T7)  [unwired: 9 in, 1 out]
          n163 = call <vilib>:"WPI_EncoderReset.vi"("EncoderDevRef"=w242) -> ("EncoderDevRef"=w241:T7)  [unwired: 9 in, 1 out]
          n164 = while {
            tunnel: w241 -> [_]
            tunnel: w239 -> [_]
            tunnel: w237 -> [w256]
            stop <- w249 stop-if-true
            n165 = call "Z900_navX_Get_YPRHfH.vi"("navX Device"=w256) -> ("YRPHfH"=w255:T11)  [unwired: 7 in, 3 out]
            n166 = call-poly <vilib>:"NT Read Value.vi"("Name"="Position") -> ("Numeric"=w246:dbl)  [unwired: 9 in, 1 out]
            n167 = case shown="Default" w246 {
              tunnel: [0.0 35.0 20.0 0.0 -20.0 -45.0] -> w247
              frame Default {
              }
              frame 1 {
              }
              frame 2 {
              }
              frame 3 {
              }
              frame 4 {
              }
              frame 5 {
              }
            }
            n168 = Unbundle By Name(w255) -> ("Yaw"=w253:dbl)  [unwired: 1 out]
            n169 = local read "Single Turn Gains"() -> (w252:T1)
            n170 = call-poly <vilib>:"PID.vi"("output range"=cluster{"output high":dbl, "output low":dbl} {"output high"=0.8, "output low"=-0.8}, "PID gains"=w252, "process variable"=w253, "setpoint"=w247) -> ("output"=w251:dbl)  [unwired: 6 in, 1 out]
            n171 = local write "Left Motor Speed"(w251) -> ()
            n172 = Multiply(x=-1.0, y=w251) -> (x*y=w250:dbl)
            n173 = local write "Right Motor Speed"(w250) -> ()
            n174 = call <vilib>:"WPI_RobotDriveRefNum Registry Get.vi"("refnum name"="Left and Right Motors") -> ("RobotDriveDevRef"=w259:T12)  [unwired: 9 in, 1 out]
            n175 = call <vilib>:"WPI_RobotDriveTankDrive.vi"("Right axis value"=w251, "Left axis value"=w250, "RobotDriveDevRef"=w259) -> ()  [unwired: 6 in, 3 out]
            n176 = call "Elapsed Time2"() -> ("Time has Elapsed"=w249:bool)  [unwired: 12 in, 7 out]
            n177 = Wait (ms)(milliseconds to wait=u32 50) -> ()  [unwired: 1 out]
          }
        }
        frame #2 {
          n178 = while {
            stop <- w277 stop-if-true
            n179 = local read "Aiming Gains"() -> (w267:T1)
            n180 = global read "Robot Global Data.vi" "T1 X"() -> (w275:dbl)
            n181 = Absolute Value(x=w275) -> (abs(x)=w280:dbl)
            n182 = Less?(x=w280, y=0.05) -> (x < y?=w278:bool)
            n183 = call-poly <vilib>:"PID.vi"("output range"=cluster{"output high":dbl, "output low":dbl} {"output high"=0.7, "output low"=-0.7}, "PID gains"=w267, "process variable"=w275, "setpoint"=0.0) -> ("output"=w269:dbl)  [unwired: 6 in, 1 out]
            n184 = case shown="False" w278 {
              tunnel: [FALSE FALSE] -> w277
              frame False {
              }
              frame True {
              }
            }
            n185 = Multiply(x=w269, y=-1.0) -> (x*y=w268:dbl)
            n186 = call <vilib>:"WPI_RobotDriveRefNum Registry Get.vi"("refnum name"="Left and Right Motors") -> ("RobotDriveDevRef"=w271:T12)  [unwired: 9 in, 1 out]
            n187 = call <vilib>:"WPI_RobotDriveTankDrive.vi"("Right axis value"=w268, "Left axis value"=w269, "RobotDriveDevRef"=w271) -> ()  [unwired: 6 in, 3 out]
            n188 = Wait (ms)(milliseconds to wait=u32 50) -> ()  [unwired: 1 out]
          }
        }
        frame #3 {
          n189 = call "Z900_navX_RefNum_Get.vi"("refnum name"="navX") -> ("navX Device"=w284:T5)  [unwired: 9 in, 1 out]
          n190 = call <vilib>:"WPI_EncoderRefNum Registry Get.vi"("refnum name"="Encoder 2") -> ("EncoderDevRef"=w286:T7)  [unwired: 9 in, 1 out]
          n191 = call <vilib>:"WPI_EncoderRefNum Registry Get.vi"("refnum name"="Encoder 1") -> ("EncoderDevRef"=w288:T7)  [unwired: 9 in, 1 out]
          n192 = call "Z900_navX_Set_ZeroYaw.vi"("navX Device"=w284) -> ("navX Device"=w283:T5)  [unwired: 9 in, 1 out]
          n193 = call <vilib>:"WPI_EncoderReset.vi"("EncoderDevRef"=w286) -> ("EncoderDevRef"=w285:T7)  [unwired: 9 in, 1 out]
          n194 = call <vilib>:"WPI_EncoderReset.vi"("EncoderDevRef"=w288) -> ("EncoderDevRef"=w287:T7)  [unwired: 9 in, 1 out]
          n195 = while {
            tunnel: w287 -> [_]
            tunnel: w285 -> [_]
            tunnel: w283 -> [w302]
            stop <- w296 stop-if-true
            n196 = call "Z900_navX_Get_YPRHfH.vi"("navX Device"=w302) -> ("YRPHfH"=w301:T11)  [unwired: 7 in, 3 out]
            n197 = call-poly <vilib>:"NT Read Value.vi"("Name"="Position") -> ("Numeric"=w293:dbl)  [unwired: 9 in, 1 out]
            n198 = case shown="Default" w293 {
              tunnel: [0.0 35.0 20.0 0.0 -20.0 -45.0] -> w294
              frame Default {
              }
              frame 1 {
              }
              frame 2 {
              }
              frame 3 {
              }
              frame 4 {
              }
              frame 5 {
              }
            }
            n199 = Unbundle By Name(w301) -> ("Yaw"=w299:dbl)  [unwired: 1 out]
            n200 = local read "Single Turn Gains"() -> (w292:T1)
            n201 = call-poly <vilib>:"PID.vi"("output range"=cluster{"output high":dbl, "output low":dbl} {"output high"=0.8, "output low"=-0.8}, "PID gains"=w292, "process variable"=w299, "setpoint"=w294) -> ("output"=w298:dbl)  [unwired: 6 in, 1 out]
            n202 = Multiply(x=-1.0, y=w298) -> (x*y=w297:dbl)
            n203 = call <vilib>:"WPI_RobotDriveRefNum Registry Get.vi"("refnum name"="Left and Right Motors") -> ("RobotDriveDevRef"=w305:T12)  [unwired: 9 in, 1 out]
            n204 = call <vilib>:"WPI_RobotDriveTankDrive.vi"("Right axis value"=w298, "Left axis value"=w297, "RobotDriveDevRef"=w305) -> ()  [unwired: 6 in, 3 out]
            n205 = call "Elapsed Time3"() -> ("Time has Elapsed"=w296:bool)  [unwired: 12 in, 7 out]
            n206 = Wait (ms)(milliseconds to wait=u32 50) -> ()  [unwired: 1 out]
          }
        }
      }
    }
    frame "New 2-Ball" {
      n207 = flat-sequence {
        frame #0 {
          w313 = u16 6 items=["Forward", "Backward", "Turn", "Shoot", "Turn Angle", "Roll G", "Roll L"] ("Task")
          n208 = call "Auton Commands.vi"("Roll"=-5.0, "Turn Angle"=0.0, "Distance"=120.0, "Task"=w313) -> ()  [unwired: 7 in]
        }
        frame #1 {
          w317 = u16 5 items=["Forward", "Backward", "Turn", "Shoot", "Turn Angle", "Roll G", "Roll L"] ("Task")
          n209 = call "Auton Commands.vi"("Roll"=-3.0, "Turn Angle"=0.0, "Distance"=120.0, "Task"=w317) -> ()  [unwired: 7 in]
        }
        frame #2 {
          w321 = u16 0 items=["Forward", "Backward", "Turn", "Shoot", "Turn Angle", "Roll G", "Roll L"] ("Task")
          n210 = call "Auton Commands.vi"("Roll"=0.0, "Turn Angle"=0.0, "Distance"=120.0, "Task"=w321) -> ()  [unwired: 7 in]
        }
        frame #3 {
          w325 = u16 2 items=["Forward", "Backward", "Turn", "Shoot", "Turn Angle", "Roll G", "Roll L"] ("Task")
          n211 = call "Auton Commands.vi"("Roll"=0.0, "Turn Angle"=0.0, "Distance"=120.0, "Task"=w325) -> ()  [unwired: 7 in]
        }
        frame #4 {
          w329 = u16 3 items=["Forward", "Backward", "Turn", "Shoot", "Turn Angle", "Roll G", "Roll L"] ("Task")
          n212 = call "Auton Commands.vi"("Roll"=0.0, "Turn Angle"=0.0, "Distance"=120.0, "Task"=w329) -> ()  [unwired: 7 in]
        }
        frame #5 {
          w333 = u16 4 items=["Forward", "Backward", "Turn", "Shoot", "Turn Angle", "Roll G", "Roll L"] ("Task")
          n213 = call "Auton Commands.vi"("Roll"=0.0, "Turn Angle"=150.0, "Distance"=120.0, "Task"=w333) -> ()  [unwired: 7 in]
        }
        frame #6 {
          w337 = u16 0 items=["Forward", "Backward", "Turn", "Shoot", "Turn Angle", "Roll G", "Roll L"] ("Task")
          n214 = call "Auton Commands.vi"("Roll"=0.0, "Turn Angle"=0.0, "Distance"=120.0, "Task"=w337) -> ()  [unwired: 7 in]
        }
        frame #7 {
          w341 = u16 6 items=["Forward", "Backward", "Turn", "Shoot", "Turn Angle", "Roll G", "Roll L"] ("Task")
          n215 = call "Auton Commands.vi"("Roll"=-5.0, "Turn Angle"=0.0, "Distance"=120.0, "Task"=w341) -> ()  [unwired: 7 in]
        }
        frame #8 {
          w345 = u16 5 items=["Forward", "Backward", "Turn", "Shoot", "Turn Angle", "Roll G", "Roll L"] ("Task")
          n216 = call "Auton Commands.vi"("Roll"=-3.0, "Turn Angle"=0.0, "Distance"=120.0, "Task"=w345) -> ()  [unwired: 7 in]
        }
        frame #9 {
          w349 = u16 0 items=["Forward", "Backward", "Turn", "Shoot", "Turn Angle", "Roll G", "Roll L"] ("Task")
          n217 = call "Auton Commands.vi"("Roll"=0.0, "Turn Angle"=0.0, "Distance"=60.0, "Task"=w349) -> ()  [unwired: 7 in]
        }
        frame #10 {
          w353 = u16 1 items=["Forward", "Backward", "Turn", "Shoot", "Turn Angle", "Roll G", "Roll L"] ("Task")
          n218 = call "Auton Commands.vi"("Roll"=0.0, "Turn Angle"=0.0, "Distance"=180.0, "Task"=w353) -> ()  [unwired: 7 in]
        }
        frame #11 {
          w357 = u16 4 items=["Forward", "Backward", "Turn", "Shoot", "Turn Angle", "Roll G", "Roll L"] ("Task")
          n219 = call "Auton Commands.vi"("Roll"=0.0, "Turn Angle"=-150.0, "Distance"=180.0, "Task"=w357) -> ()  [unwired: 7 in]
        }
        frame #12 {
          w361 = u16 3 items=["Forward", "Backward", "Turn", "Shoot", "Turn Angle", "Roll G", "Roll L"] ("Task")
          n220 = call "Auton Commands.vi"("Roll"=0.0, "Turn Angle"=-150.0, "Distance"=180.0, "Task"=w361) -> ()  [unwired: 7 in]
        }
      }
    }
    frame "Drive + Shoot" {
      n221 = call "Z900_navX_RefNum_Get.vi"("refnum name"="navX") -> ("navX Device"=w373:T5)  [unwired: 9 in, 1 out]
      n222 = call <vilib>:"WPI_EncoderRefNum Registry Get.vi"("refnum name"="Encoder 2") -> ("EncoderDevRef"=w371:T7)  [unwired: 9 in, 1 out]
      n223 = call <vilib>:"WPI_EncoderRefNum Registry Get.vi"("refnum name"="Encoder 1") -> ("EncoderDevRef"=w369:T7)  [unwired: 9 in, 1 out]
      n224 = call "Z900_navX_Set_ZeroYaw.vi"("navX Device"=w373) -> ("navX Device"=w374:T5)  [unwired: 9 in, 1 out]
      n225 = call <vilib>:"WPI_EncoderReset.vi"("EncoderDevRef"=w371) -> ("EncoderDevRef"=w372:T7)  [unwired: 9 in, 1 out]
      n226 = call <vilib>:"WPI_EncoderReset.vi"("EncoderDevRef"=w369) -> ("EncoderDevRef"=w370:T7)  [unwired: 9 in, 1 out]
      n227 = flat-sequence {
        tunnel: w374 -> [w378]
        tunnel: w372 -> [w377]
        tunnel: w370 -> [w376]
        tunnel: w365 -> [w375]
        frame #0 {
          n228 = while {
            tunnel: w376 -> [w416]
            tunnel: w377 -> [w415]
            tunnel: w378 -> [w414]
            tunnel: w375 -> [w384]
            stop <- w385 stop-if-true
            n229 = call <vilib>:"WPI_EncoderGet.vi"("EncoderDevRef"=w415) -> ("Distance"=w391:dbl, "Rate"=→"E2 Rate":dbl)  [unwired: 5 in, 4 out]
            n230 = call-poly <vilib>:"NT Read Value.vi"("Name"=w384) -> ("Numeric"=w383:dbl)  [unwired: 9 in, 1 out]
            n231 = call "Z900_navX_Get_YPRHfH.vi"("navX Device"=w414) -> ("YRPHfH"=w417:T11)  [unwired: 7 in, 3 out]
            n232 = Divide(x=w383, y=100.0) -> (x/y=w381:dbl)
            n233 = call <vilib>:"WPI_EncoderGet.vi"("EncoderDevRef"=w416) -> ("Distance"=w392:dbl, "Rate"=→"E1 Rate":dbl)  [unwired: 5 in, 4 out]
            n234 = Bundle(w381, "output low"=0.15) -> (w379:cluster{dbl, "output low":dbl})  [unwired: 1 in]
            n235 = Unbundle By Name(w417) -> ("Yaw"=w393:dbl)  [unwired: 1 out]
            "Yaw" <- w393
            n236 = call-poly <vilib>:"NT Write Value.vi"("Numeric"=w391, "Name"="E2 Dist") -> ()  [unwired: 9 in, 1 out]
            n237 = local read "Distance"() -> (w401:dbl)
            n238 = call-poly <vilib>:"NT Write Value.vi"("Numeric"=w392, "Name"="E1 Dist") -> ()  [unwired: 9 in, 1 out]
            n239 = Multiply(x=w401, y=13.7) -> (x*y=w390:dbl)
            n240 = local read "Speed Gains"() -> (w395:T1)
            n241 = local read "Yaw"() -> (w399:T1)
            n242 = Add(x=w392, y=w391) -> (x+y=w413:dbl)
            n243 = Divide(x=w413, y=2.0) -> (x/y=w389:dbl)
            n244 = Subtract(x=w390, y=w389) -> (x-y=w388:dbl)
            n245 = Absolute Value(x=w388) -> (abs(x)=w387:dbl)
            n246 = Less?(x=w387, y=30.0) -> (x < y?=w385:bool)
            n247 = call-poly <vilib>:"PID.vi"("output range"=cluster{"output high":dbl, "output low":dbl} {"output high"=0.2, "output low"=-0.2}, "PID gains"=w399, "process variable"=w393, "setpoint"=0.0) -> ("output"=w406:dbl)  [unwired: 6 in, 1 out]
            n248 = call-poly <vilib>:"PID.vi"("output range"=w379, "PID gains"=w395, "process variable"=w389, "setpoint"=w390) -> ("output"=w403:dbl)  [unwired: 6 in, 1 out]
            n249 = Multiply(x=-1.0, y=w406) -> (x*y=w407:dbl)
            n250 = Add(x=1.0, y=w407) -> (x+y=w408:dbl)
            n251 = Wait (ms)(milliseconds to wait=u32 50) -> ()  [unwired: 1 out]
            n252 = Add(x=w406, y=1.0) -> (x+y=w409:dbl)
            n253 = Multiply(x=w403, y=w408) -> (x*y=w396:dbl)
            n254 = Multiply(x=w403, y=w409) -> (x*y=w398:dbl)
            n255 = call <vilib>:"WPI_RobotDriveRefNum Registry Get.vi"("refnum name"="Left and Right Motors") -> ("RobotDriveDevRef"=w419:T12)  [unwired: 9 in, 1 out]
            n256 = call <vilib>:"WPI_RobotDriveTankDrive.vi"("Right axis value"=w398, "Left axis value"=w396, "RobotDriveDevRef"=w419) -> ()  [unwired: 6 in, 3 out]
            n257 = local write "Right Motor Speed"(w398) -> ()
            n258 = local write "Left Motor Speed"(w396) -> ()
          }
        }
        frame #1 {
          n259 = call "Z900_navX_RefNum_Get.vi"("refnum name"="navX") -> ("navX Device"=w424:T5)  [unwired: 9 in, 1 out]
          n260 = call <vilib>:"WPI_EncoderRefNum Registry Get.vi"("refnum name"="Encoder 2") -> ("EncoderDevRef"=w426:T7)  [unwired: 9 in, 1 out]
          n261 = call <vilib>:"WPI_EncoderRefNum Registry Get.vi"("refnum name"="Encoder 1") -> ("EncoderDevRef"=w428:T7)  [unwired: 9 in, 1 out]
          n262 = call "Z900_navX_Set_ZeroYaw.vi"("navX Device"=w424) -> ("navX Device"=w423:T5)  [unwired: 9 in, 1 out]
          n263 = call <vilib>:"WPI_EncoderReset.vi"("EncoderDevRef"=w426) -> ("EncoderDevRef"=w425:T7)  [unwired: 9 in, 1 out]
          n264 = call <vilib>:"WPI_EncoderReset.vi"("EncoderDevRef"=w428) -> ("EncoderDevRef"=w427:T7)  [unwired: 9 in, 1 out]
          n265 = while {
            tunnel: w427 -> [_]
            tunnel: w425 -> [_]
            tunnel: w423 -> [w442]
            stop <- w435 stop-if-true
            n266 = call "Z900_navX_Get_YPRHfH.vi"("navX Device"=w442) -> ("YRPHfH"=w441:T11)  [unwired: 7 in, 3 out]
            n267 = call-poly <vilib>:"NT Read Value.vi"("Name"="Position") -> ("Numeric"=w432:dbl)  [unwired: 9 in, 1 out]
            n268 = case shown="Default" w432 {
              tunnel: [0.0 35.0 20.0 0.0 -20.0 -45.0] -> w433
              frame Default {
              }
              frame 1 {
              }
              frame 2 {
              }
              frame 3 {
              }
              frame 4 {
              }
              frame 5 {
              }
            }
            n269 = Unbundle By Name(w441) -> ("Yaw"=w439:dbl)  [unwired: 1 out]
            n270 = local read "Single Turn Gains"() -> (w438:T1)
            n271 = call-poly <vilib>:"PID.vi"("output range"=cluster{"output high":dbl, "output low":dbl} {"output high"=0.8, "output low"=-0.8}, "PID gains"=w438, "process variable"=w439, "setpoint"=w433) -> ("output"=w437:dbl)  [unwired: 6 in, 1 out]
            n272 = local write "Left Motor Speed"(w437) -> ()
            n273 = Multiply(x=-1.0, y=w437) -> (x*y=w436:dbl)
            n274 = local write "Right Motor Speed"(w436) -> ()
            n275 = call <vilib>:"WPI_RobotDriveRefNum Registry Get.vi"("refnum name"="Left and Right Motors") -> ("RobotDriveDevRef"=w445:T12)  [unwired: 9 in, 1 out]
            n276 = call <vilib>:"WPI_RobotDriveTankDrive.vi"("Right axis value"=w437, "Left axis value"=w436, "RobotDriveDevRef"=w445) -> ()  [unwired: 6 in, 3 out]
            n277 = call "Elapsed Time"() -> ("Time has Elapsed"=w435:bool)  [unwired: 12 in, 7 out]
            n278 = Wait (ms)(milliseconds to wait=u32 50) -> ()  [unwired: 1 out]
          }
        }
        frame #2 {
          n279 = while {
            stop <- w463 stop-if-true
            n280 = local read "Aiming Gains"() -> (w453:T1)
            n281 = global read "Robot Global Data.vi" "T1 X"() -> (w461:dbl)
            n282 = Absolute Value(x=w461) -> (abs(x)=w466:dbl)
            n283 = Less?(x=w466, y=0.05) -> (x < y?=w464:bool)
            n284 = call-poly <vilib>:"PID.vi"("output range"=cluster{"output high":dbl, "output low":dbl} {"output high"=0.7, "output low"=-0.7}, "PID gains"=w453, "process variable"=w461, "setpoint"=0.0) -> ("output"=w455:dbl)  [unwired: 6 in, 1 out]
            n285 = case shown="False" w464 {
              tunnel: [FALSE FALSE] -> w463
              frame False {
              }
              frame True {
              }
            }
            n286 = Multiply(x=w455, y=-1.0) -> (x*y=w454:dbl)
            n287 = call <vilib>:"WPI_RobotDriveRefNum Registry Get.vi"("refnum name"="Left and Right Motors") -> ("RobotDriveDevRef"=w457:T12)  [unwired: 9 in, 1 out]
            n288 = call <vilib>:"WPI_RobotDriveTankDrive.vi"("Right axis value"=w454, "Left axis value"=w455, "RobotDriveDevRef"=w457) -> ()  [unwired: 6 in, 3 out]
            n289 = Wait (ms)(milliseconds to wait=u32 50) -> ()  [unwired: 1 out]
          }
        }
      }
    }
    frame "Dashboard Auton" {
      n290 = flat-sequence {
        frame #0 {
          n291 = while {
            stop <- w494 stop-if-true
            n292 = global read "Robot Global Data.vi" "T1 X"() -> (w492:dbl)
            n293 = Absolute Value(x=w492) -> (abs(x)=w497:dbl)
            n294 = Less?(x=w497, y=0.125) -> (x < y?=w495:bool)
            n295 = call-poly <vilib>:"PID.vi"("output range"=cluster{"output high":dbl, "output low":dbl} {"output high"=0.2, "output low"=-0.2}, "PID gains"="Aiming Gains", "process variable"=w492, "setpoint"=0.1) -> ("output"=w487:dbl)  [unwired: 6 in, 1 out]
            n296 = case shown="True" w495 {
              tunnel: [FALSE TRUE] -> w494
              frame False {
              }
              frame True {
              }
            }
            n297 = Multiply(x=w487, y=1.0) -> (x*y=w474:dbl)
            n298 = call <vilib>:"WPI_MotorControlRefNum Registry Get.vi"("refnum name"="Turret") -> ("error out"=w486:errorcluster, "MotorControlDevRef"=w475:T13)  [unwired: 9 in]
            n299 = call <vilib>:"WPI_CANTalonSRX_ConfigEnabledLimits.vi"("CAN Talon SRX Ref"=w475, "Forward Soft Limit Enable"=TRUE, "Reverse Soft Limit Enable"=TRUE) -> ("CAN Talon SRX Ref"=w483:T13, "error out"=w482:errorcluster)  [unwired: 11 in]
            n300 = call <vilib>:"WPI_CANTalonSRX_ConfigSoftLimits.vi"("CAN Talon SRX Ref"=w483, "Forward Limit Position"=1.4, "Reverse Limit Position"=0.2, "error in (no error)"=w482) -> ("CAN Talon SRX Ref"=w478:T13, "error out"=w479:errorcluster)  [unwired: 10 in]
            n301 = call <vilib>:"WPI_CANTalonSRX_ConfigBrakeCoast.vi"("error in (no error)"=w479, "Brake / Coast Mode"=WPI_CANTalonSRX_BrakeOverride."Override to Brake", "CAN Talon SRX Ref"=w478) -> ("error out"=w473:errorcluster, "CAN Talon SRX Ref"=w472:T13)  [unwired: 7 in]
            n302 = call <vilib>:"WPI_MotorControlSetOutput.vi"("error in (no error)"=w486, "Output"=w474, "MotorControlDevRef"=w472) -> ()  [unwired: 6 in, 3 out]
            n303 = call <vilib>:"WPI_CANTalonSRX_GetStatus.vi"("error in (no error)"=w473, "CAN Talon SRX Ref"=w472) -> ("Talon SRX Status"=w471:T20)  [unwired: 7 in, 2 out]
            n304 = Unbundle By Name(w471) -> ("Encoder Position"=w470:dbl)
            n305 = call-poly <vilib>:"NT Write Value.vi"("Numeric"=w470, "Name"="Encoder") -> ()  [unwired: 9 in, 1 out]
            n306 = Wait (ms)(milliseconds to wait=u32 50) -> ()  [unwired: 1 out]
          }
        }
        frame #1 {
          n307 = while {
            stop <- w529 stop-if-true
            n308 = local read "Aiming Gains"() -> (w501:T1)
            n309 = global read "Robot Global Data.vi" "T1 X"() -> (w527:dbl)
            n310 = Absolute Value(x=w527) -> (abs(x)=w532:dbl)
            n311 = Less?(x=w532, y=0.125) -> (x < y?=w530:bool)
            n312 = call-poly <vilib>:"PID.vi"("output range"=cluster{"output high":dbl, "output low":dbl} {"output high"=0.2, "output low"=-0.2}, "PID gains"=w501, "process variable"=w527, "setpoint"=0.1) -> ("output"=w523:dbl)  [unwired: 6 in, 1 out]
            n313 = case shown="True" w530 {
              tunnel: [FALSE FALSE] -> w529
              frame False {
              }
              frame True {
              }
            }
            n314 = Multiply(x=w523, y=1.0) -> (x*y=w510:dbl)
            n315 = call <vilib>:"WPI_MotorControlRefNum Registry Get.vi"("refnum name"="Turret") -> ("error out"=w522:errorcluster, "MotorControlDevRef"=w511:T13)  [unwired: 9 in]
            n316 = global read "Robot Global Data.vi" "RPM"() -> (w500:dbl)
            n317 = call <vilib>:"WPI_CANTalonSRX_ConfigEnabledLimits.vi"("CAN Talon SRX Ref"=w511, "Forward Soft Limit Enable"=TRUE, "Reverse Soft Limit Enable"=TRUE) -> ("CAN Talon SRX Ref"=w519:T13, "error out"=w518:errorcluster)  [unwired: 11 in]
            n318 = call <vilib>:"WPI_MotorControlRefNum Registry Get.vi"("refnum name"="Shooter") -> ("error out"=w504:errorcluster, "MotorControlDevRef"=w503:T13)  [unwired: 9 in]
            n319 = call <vilib>:"WPI_CANTalonSRX_ConfigSoftLimits.vi"("CAN Talon SRX Ref"=w519, "Forward Limit Position"=1.4, "Reverse Limit Position"=0.2, "error in (no error)"=w518) -> ("CAN Talon SRX Ref"=w514:T13, "error out"=w515:errorcluster)  [unwired: 10 in]
            n320 = call <vilib>:"WPI_CANTalonSRX_ConfigBrakeCoast.vi"("error in (no error)"=w515, "Brake / Coast Mode"=WPI_CANTalonSRX_BrakeOverride."Override to Brake", "CAN Talon SRX Ref"=w514) -> ("error out"=w509:errorcluster, "CAN Talon SRX Ref"=w508:T13)  [unwired: 7 in]
            n321 = call <vilib>:"WPI_MotorControlSetOutput.vi"("error in (no error)"=w522, "Output"=w510, "MotorControlDevRef"=w508) -> ()  [unwired: 6 in, 3 out]
            n322 = call <vilib>:"WPI_MotorControlSetOutput.vi"("error in (no error)"=w504, "Output"=w500, "MotorControlDevRef"=w503) -> ()  [unwired: 6 in, 3 out]
            n323 = call <vilib>:"WPI_CANTalonSRX_GetStatus.vi"("error in (no error)"=w509, "CAN Talon SRX Ref"=w508) -> ("Talon SRX Status"=w507:T20)  [unwired: 7 in, 2 out]
            n324 = Unbundle By Name(w507) -> ("Encoder Position"=w506:dbl)
            n325 = call-poly <vilib>:"NT Write Value.vi"("Numeric"=w506, "Name"="Encoder") -> ()  [unwired: 9 in, 1 out]
            n326 = Wait (ms)(milliseconds to wait=u32 50) -> ()  [unwired: 1 out]
          }
        }
      }
    }
  }
